vi "index Values of R.vi"() -> ()   [LabVIEW 2022 SP3]
panel:
  in  "index values of R":i32[](array[numeric])
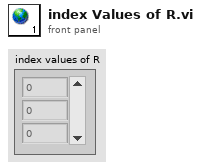
[diagram p1: front panel]
diagram:
